vi "反色计算.vi"(11 "颜色盒":u32(colorbox)) -> (3 "反色":u32(colorbox) caption="颜色")   [LabVIEW 2013]
panel:
  in  "G 2":u8 caption="G"
  in  "R 2":u8 caption="R"
  in  "B 2":u8 caption="B"
  out "B":u8
  out "R":u8
  out "G":u8
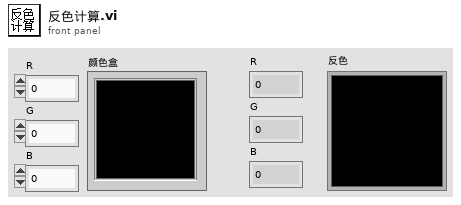
[diagram p1: front panel]
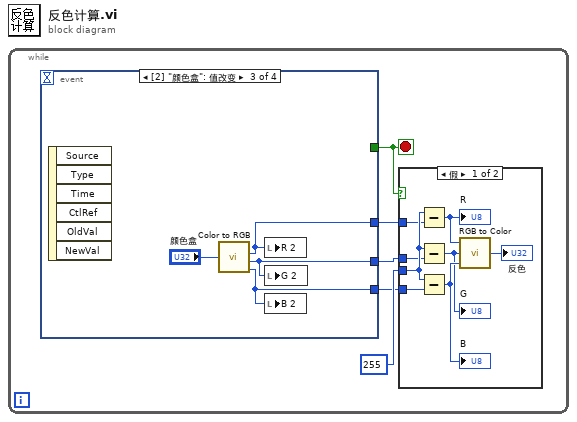
[diagram p0: block diagram]
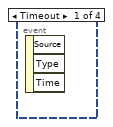
[diagram p3: hidden frame]
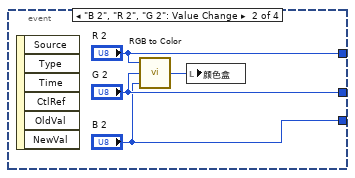
[diagram p4: hidden frame]
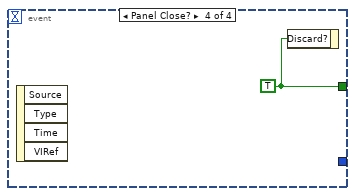
[diagram p5: hidden frame]
diagram:
  n1 = while {
    stop <- w1 stop-if-true
    n2 = event shown="[2] \"颜色盒\": 值改变" {
      selector: _ -> [_ _ _ _]
      dyn-events: _ -> [_ _ _ _]
      timeout: _ -> [_ _ _ _]
      tunnel: [_ "R 2" w20 _] -> w4
      tunnel: [_ "G 2" w19 _] -> w3
      tunnel: [_ "B 2" w18 _] -> w2
      tunnel: [_ _ _ w22] -> w1
      event Timeout {
        n3 = event-data() -> ()  [unwired: 1 in, 3 out]
      }
      event "B 2", "R 2", "G 2": Value Change {
        n4 = event-data() -> ()  [unwired: 1 in, 6 out]
        n5 = call <vilib>:"RGB to Color.vi"("B"="B 2", "G"="G 2", "R"="R 2") -> ("Color"=w17:u32)
        n6 = local write "颜色盒"(w17) -> ()
      }
      event "颜色盒": Value Change {
        n7 = event-data() -> ()  [unwired: 1 in, 6 out]
        n8 = call <vilib>:"Color to RGB.vi"("Color"="颜色盒") -> ("R"=w20:u8, "G"=w19:u8, "B"=w18:u8)  [unwired: 1 out]
        n9 = local write "R 2"(w20) -> ()
        n10 = local write "G 2"(w19) -> ()
        n11 = local write "B 2"(w18) -> ()
      }
      event Panel Close? {
        w22 = TRUE ("放弃？")
        n12 = event-data() -> ()  [unwired: 1 in, 4 out]
        n13 = event-data("Discard?"=w22) -> ()  [unwired: 1 in, 1 out]
      }
    }
    n14 = case shown="假" w1 {
      tunnel: u8 255 -> [w9 _]
      tunnel: w4 -> [w8 _]
      tunnel: w3 -> [w7 _]
      tunnel: w2 -> [w6 _]
      frame False {
        n15 = Subtract(x=w9, y=w8) -> (x-y=w11:u8)
        "R" <- w11
        n16 = Subtract(x=w9, y=w7) -> (x-y=w12:u8)
        "G" <- w12
        n17 = Subtract(x=w9, y=w6) -> (x-y=w13:u8)
        "B" <- w13
        n18 = call <vilib>:"RGB to Color.vi"("B"=w13, "G"=w12, "R"=w11) -> ("Color"=→"反色":u32)
      }
      frame True {
      }
    }
  }
